vi "TfidfVectorizer.vi"(8 "error in":errorcluster caption="entrée d'erreur", 11 "TfidfVectorizer":T1={"encoding"="utf-8", "decode_error"="strict", "strip_accents"="None", "lowercase"=TRUE, "preprocessor"="None", "tokenizer"="None", "analyzer"="word", "stop_words"={"Type"="None", "list"=[]}, "token_pattern"="(?u)\\b\\w\\w+\\b", "ngram_range"={"min_n"=1, "max_n"=1}, "max_df"=1.0, "min_df"=1.0, "max_features"=-1, "vocabulary"={"Clé"=["None"], "Valeur"=[]}, "binary"=FALSE, "dtype"="float", "norm"="l2", "use_idf"=TRUE, "smooth_idf"=TRUE, "sublinear_tf"=FALSE} {"max_features" min=-1; "min_df" min=0.0 max=1.0; "max_df" min=0.0 max=1.0}) -> (0 "error out":errorcluster caption="sortie d'erreur", 3 "TfidfVectorizer.lvclass":refnum<class "TfidfVectorizer.lvclass">)   [LabVIEW 2020]
doc: "Convert a collection of raw documents to a matrix of TF-IDF features.\n\nEquivalent to CountVectorizer followed by TfidfTransformer.\n\nParameters :\n\n- encoding : str, default=’utf-8’\nIf bytes or files are given to analyze, this encoding is used to decode.\n\n- decode_error : {‘strict’, ‘ignore’, ‘replace’}, default=’strict’\nInstruction on what to do if a byte sequence is given to analyze that contains characters not of the given encoding. By default, it is ‘strict’, meaning that a UnicodeDecodeError will be raised. Other values are ‘ignore’ and ‘replace’.\n\n- strip_accents : {‘ascii’, ‘unicode’}, default=None\nRemove accents and perform other character normalization during the preprocessing step. ‘ascii’ is a fast method that only works on characters that have an direct ASCII mapping. ‘unicode’ is a slightly slower method that works on any characters. None (default) does nothing.\n\nBoth ‘ascii’ and ‘unicode’ use NFKD normalization from unicodedata.normalize.\n\n- lowercase : bool, default=True\nConvert all characters to lowercase before tokenizing.\n\n- preprocessor : callable, default=None\nOverride the preprocessing (string transformation) stage while preserving the tokenizing and n-grams generation steps. Only applies if analyzer is not callable.\n\n- tokenizer : callable, default=None\nOverride the string tokenization step while preserving the preprocessing and n-grams generation steps. Only applies if analyzer == 'word'.\n\n- analyzer : {‘word’, ‘char’, ‘char_wb’} or callable, default=’word’\nWhether the feature should be made of word or character n-grams. Option ‘char_wb’ creates character n-grams only from text inside word boundaries; n-grams at the edges of words are padded with space.\n\nIf a callable is passed it is used to extract the sequence of features out of the raw, unprocessed input.\n\n- stop_words : {‘english’}, list, default=None\nIf a string, it is passed to _check_stop_list and the appropriate stop list is returned. ‘english’ is currently the only supported string value. There are several known issues with ‘english’ and you should consider an alternative (see Using stop words).\n\nIf a list, that list is assumed to contain stop words, all of which will be removed from the resulting tokens. Only applies if analyzer == 'word'.\n\nIf None, no stop words will be used. max_df can be set to a value in the range [0.7, 1.0) to automatically detect and filter stop words based on intra corpus document frequency of terms.\n\n- token_pattern : str\nRegular expression denoting what constitutes a “token”, only used if analyzer == 'word'. The default regexp selects tokens of 2 or more alphanumeric characters (punctuation is completely ignored and always treated as a token separator).\n\n- ngram_range : tuple (min_n, max_n), default=(1, 1)\nThe lower and upper boundary of the range of n-values for different n-grams to be extracted. All values of n such that min_n <= n <= max_n will be used. For example an ngram_range of (1, 1) means only unigrams, (1, 2) means unigrams and bigrams, and (2, 2) means only bigrams. Only applies if analyzer is not callable.\n\n- max_df : float or int, default=1.0\nWhen building the vocabulary ignore terms that have a document frequency strictly higher than the given threshold (corpus-specific stop words). If float in range [0.0, 1.0], the parameter represents a proportion of documents, integer absolute counts. This parameter is ignored if vocabulary is not None.\n\n- min_df : float or int, default=1\nWhen building the vocabulary ignore terms that have a document frequency strictly lower than the given threshold. This value is also called cut-off in the literature. If float in range of [0.0, 1.0], the parameter represents a proportion of documents, integer absolute counts. This parameter is ignored if vocabulary is not None.\n\n- max_features : int, default=None\nIf not None, build a vocabulary that only consider the top max_features ordered by term frequency across the corpus.\n\nThis parameter is ignored if vocabulary is not None.\n\n- vocabulary : Mapping or iterable, default=None\nEither a Mapping (e.g., a dict) where keys are terms and values are indices in the feature matrix, or an iterable over terms. If not given, a vocabulary is determined from the input documents.\n\n- binary : bool, default=False\nIf True, all non-zero term counts are set to 1. This does not mean outputs will have only 0/1 values, only that the tf term in tf-idf is binary. (Set idf and normalization to False to get 0/1 outputs).\n\n- dtype : dtype, default=float64\nType of the matrix returned by fit_transform() or transform().\n\n- norm : {‘l1’, ‘l2’}, default=’l2’\nEach output row will have unit norm, either: * ‘l2’: Sum of squares of vector elements is 1. The cosine similarity between two vectors is their dot product when l2 norm has been applied. * ‘l1’: Sum of absolute values of vector elements is 1. See preprocessing.normalize.\n\n- use_idf : bool, default=True\nEnable inverse-document-frequency reweighting.\n\n- smooth_idf : bool, default=True\nSmooth idf weights by adding one to document frequencies, as if an extra document was seen containing every term in the collection exactly once. Prevents zero divisions.\n\n- sublinear_tf : bool, default=False\nApply sublinear tf scaling, i.e. replace tf with 1 + log(tf).\n\n\n\nMethods :"
uses:
  TfidfVectorizer.lvclass
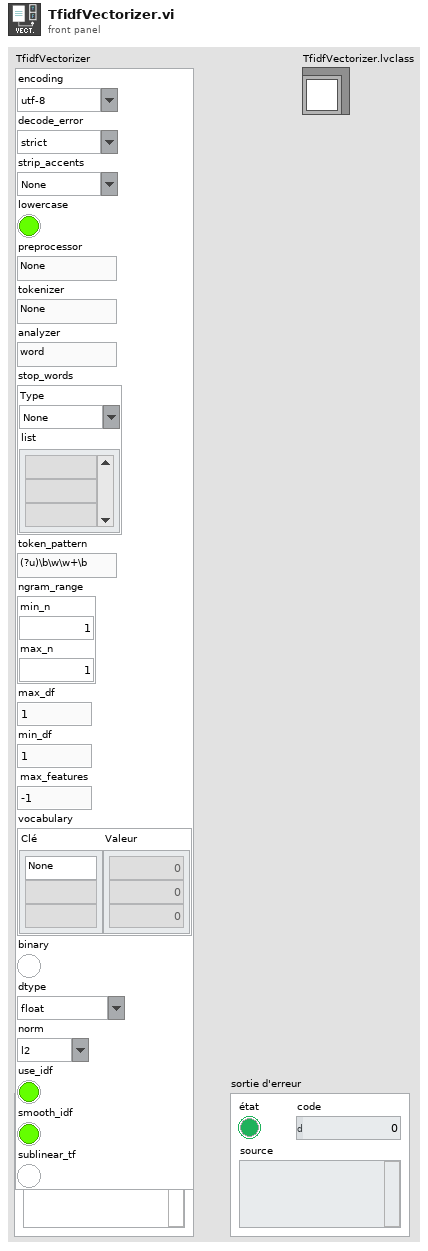
[diagram p1: front panel]
types:
  T1 = cluster{"encoding":string, "decode_error":string, "strip_accents":string, "lowercase":bool, "preprocessor":string, "tokenizer":string, "analyzer":string, "stop_words":cluster{"Type":string, "list":string[]}, "token_pattern":string, "ngram_range":cluster{"min_n":i32, "max_n":i32}, "max_df":dbl, "min_df":dbl, "max_features":i32, "vocabulary":cluster{"Clé":string[], "Valeur":i32[]}, "binary":bool, "dtype":string, "norm":string, "use_idf":bool, "smooth_idf":bool, "sublinear_tf":bool}
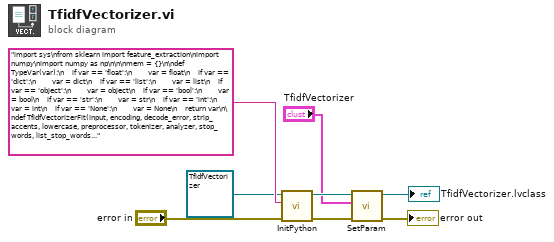
[diagram p0: block diagram]
diagram:
  n1 = call-dynamic "InitPython.vi"("error in (no error)"="error in", "Python Instruction"="import sys\nfrom sklearn import feature_extraction\nimport numpy\nimport numpy as np\n\n\nmem = {}\n\ndef TypeVar(var):\n    if var == 'float':\n        var = float\n    if var == 'dict':\n        var = dict\n    if var == 'list':\n        var = list\n    if var == 'object':\n        var = object\n    if var == 'bool':\n        var = bool\n    if var == 'str':\n        var = str\n    if var == 'int':\n        var = int\n    if var == 'None':\n        var = None\n    return var\n\ndef TfidfVectorizerFit(input, encoding, decode_error, strip_accents, lowercase, preprocessor, tokenizer, analyzer, stop_words, list_stop_words, token_pattern, min_n, max_n, max_df, min_df, max_features, vocabulary, binary, dtype, norm, use_idf, smooth_idf, sublinear_tf, X, doc):\n    X = eval(X)\n    dtype = TypeVar(dtype) \n    list_analyzer = ['word', 'char', 'char_wb']\n    if tokenizer == 'None' or tokenizer == '':\n        tokenizer = None\n    else:\n        tokenizer = eval(tokenizer)\n    if preprocessor == 'None' or preprocessor == '':\n        preprocessor = None\n    else:\n        preprocessor = eval(preprocessor)\n    if strip_accents == 'None':\n        strip_accents = None\n    if stop_words == 'None':\n        stop_words = None\n    elif stop_words == 'list':\n        stop_words = list_stop_words\n    else: \n        pass\n    if norm == 'None':\n        norm = None\n    if max_features == -1:\n        max_features = None\n    if vocabulary == 'None':\n        vocabulary = None\n    else:\n        vocabulary = eval(vocabulary)\n    if analyzer not in list_analyzer:\n        analyzer = eval(analyzer) \n    try:\n        TfidfVectorizer = feature_extraction.text.TfidfVectorizer(input, encoding, decode_error, strip_accents, lowercase, preprocessor, tokenizer, analyzer, stop_words, token_pattern, (min_n, max_n), max_df, min_df, max_features, vocabulary, binary, dtype, norm, use_idf, smooth_idf, sublinear_tf).fit(X)\n        mem['FitTfidfVectorizer'] = TfidfVectorizer\n        return str('OK')\n    except:\n        erreur = sys.exc_info()\n        typerr = u\"%s\" % (erreur[0])\n        typerr = typerr[typerr.find(\"'\")+1:typerr.rfind(\"'\")]\n        msgerr = u\"%s\" % (erreur[1])\n        message = str('/!\\\\ {0} : {1}'. format(typerr,msgerr))\n        return message \n\ndef TfidfVectorizerFitTransform(input, encoding, decode_error, strip_accents, lowercase, preprocessor, tokenizer, analyzer, stop_words, list_stop_words, token_pattern, min_n, max_n, max_df, min_df, max_features, vocabulary, binary, dtype, norm, use_idf, smooth_idf, sublinear_tf, X, doc):\n    X = eval(X)\n    dtype = TypeVar(dtype) \n    list_analyzer = ['word', 'char', 'char_wb']\n    if tokenizer == 'None' or tokenizer == '':\n        tokenizer = None\n    else:\n        tokenizer = eval(tokenizer)\n    if preprocessor == 'None' or preprocessor == '':\n        preprocessor = None\n    else:\n        preprocessor = eval(preprocessor)\n    if strip_accents == 'None':\n        strip_accents = None\n    if stop_words == 'None':\n        stop_words = None\n    elif stop_words == 'list':\n        stop_words = list_stop_words\n    else: \n        pass\n    if norm == 'None':\n        norm = None\n    if max_features == -1:\n        max_features = None\n    if vocabulary == 'None':\n        vocabulary = None\n    else:\n        vocabulary = eval(vocabulary)\n    if analyzer not in list_analyzer:\n        analyzer = eval(analyzer) \n    try:\n        TfidfVectorizer = feature_extraction.text.TfidfVectorizer(input, encoding, decode_error, strip_accents, lowercase, preprocessor, tokenizer, analyzer, stop_words, token_pattern, (min_n, max_n), max_df, min_df, max_features, vocabulary, binary, dtype, norm, use_idf, smooth_idf, sublinear_tf).fit_transform(X)\n        Mat = TfidfVectorizer.tocoo()\n        return str(list(zip(Mat.row, Mat.col, Mat.data)))\n    except:\n        erreur = sys.exc_info()\n        typerr = u\"%s\" % (erreur[0])\n        typerr = typerr[typerr.find(\"'\")+1:typerr.rfind(\"'\")]\n        msgerr = u\"%s\" % (erreur[1])\n        message = str('/!\\\\ {0} : {1}'. format(typerr,msgerr))\n        return message \n    \ndef TfidfVectorizerTransform(input, encoding, decode_error, strip_accents, lowercase, preprocessor, tokenizer, analyzer, stop_words, list_stop_words, token_pattern, min_n, max_n, max_df, min_df, max_features, vocabulary, binary, dtype, norm, use_idf, smooth_idf, sublinear_tf, X, doc):\n    X = eval(X)\n    dtype = TypeVar(dtype) \n    list_analyzer = ['word', 'char', 'char_wb']\n    if tokenizer == 'None' or tokenizer == '':\n        tokenizer = None\n    else:\n        tokenizer = eval(tokenizer)\n    if preprocessor == 'None' or preprocessor == '':\n        preprocessor = None\n    else:\n        preprocessor = eval(preprocessor)\n    if strip_accents == 'None':\n        strip_accents = None\n    if stop_words == 'None':\n        stop_words = None\n    elif stop_words == 'list':\n        stop_words = list_stop_words\n    else: \n        pass\n    if norm == 'None':\n        norm = None\n    if max_features == -1:\n        max_features = None\n    if vocabulary == 'None':\n        vocabulary = None\n    else:\n        vocabulary = eval(vocabulary)\n    if analyzer not in list_analyzer:\n        analyzer = eval(analyzer) \n    try:\n        TfidfVectorizer = mem['FitTfidfVectorizer'].transform(X)\n        Mat = TfidfVectorizer.tocoo()\n        return str(list(zip(Mat.row, Mat.col, Mat.data)))\n    except:\n        erreur = sys.exc_info()\n        typerr = u\"%s\" % (erreur[0])\n        typerr = typerr[typerr.find(\"'\")+1:typerr.rfind(\"'\")]\n        msgerr = u\"%s\" % (erreur[1])\n        message = str('/!\\\\ {0} : {1}'. format(typerr,msgerr))\n        return message\n    \ndef TfidfVectorizerDecode(input, encoding, decode_error, strip_accents, lowercase, preprocessor, tokenizer, analyzer, stop_words, list_stop_words, token_pattern, min_n, max_n, max_df, min_df, max_features, vocabulary, binary, dtype, norm, use_idf, smooth_idf, sublinear_tf, X, doc):\n    X = eval(X)\n    dtype = TypeVar(dtype) \n    list_analyzer = ['word', 'char', 'char_wb']\n    if tokenizer == 'None' or tokenizer == '':\n        tokenizer = None\n    else:\n        tokenizer = eval(tokenizer)\n    if preprocessor == 'None' or preprocessor == '':\n        preprocessor = None\n    else:\n        preprocessor = eval(preprocessor)\n    if strip_accents == 'None':\n        strip_accents = None\n    if stop_words == 'None':\n        stop_words = None\n    elif stop_words == 'list':\n        stop_words = list_stop_words\n    else: \n        pass\n    if norm == 'None':\n        norm = None\n    if max_features == -1:\n        max_features = None\n    if vocabulary == 'None':\n        vocabulary = None\n    else:\n        vocabulary = eval(vocabulary)\n    if analyzer not in list_analyzer:\n        analyzer = eval(analyzer) \n    try:\n        TfidfVectorizer = feature_extraction.text.TfidfVectorizer(input, encoding, decode_error, strip_accents, lowercase, preprocessor, tokenizer, analyzer, stop_words, token_pattern, (min_n, max_n), max_df, min_df, max_features, vocabulary, binary, dtype, norm, use_idf, smooth_idf, sublinear_tf).decode(doc)\n        return str(TfidfVectorizer)\n    except:\n        erreur = sys.exc_info()\n        typerr = u\"%s\" % (erreur[0])\n        typerr = typerr[typerr.find(\"'\")+1:typerr.rfind(\"'\")]\n        msgerr = u\"%s\" % (erreur[1])\n        message = str('/!\\\\ {0} : {1}'. format(typerr,msgerr))\n        return message\n    \ndef TfidfVectorizerFeatNames(input, encoding, decode_error, strip_accents, lowercase, preprocessor, tokenizer, analyzer, stop_words, list_stop_words, token_pattern, min_n, max_n, max_df, min_df, max_features, vocabulary, binary, dtype, norm, use_idf, smooth_idf, sublinear_tf, X, doc):\n    X = eval(X)\n    dtype = TypeVar(dtype) \n    list_analyzer = ['word', 'char', 'char_wb']\n    if tokenizer == 'None' or tokenizer == '':\n        tokenizer = None\n    else:\n        tokenizer = eval(tokenizer)\n    if preprocessor == 'None' or preprocessor == '':\n        preprocessor = None\n    else:\n        preprocessor = eval(preprocessor)\n    if strip_accents == 'None':\n        strip_accents = None\n    if stop_words == 'None':\n        stop_words = None\n    elif stop_words == 'list':\n        stop_words = list_stop_words\n    else: \n        pass\n    if norm == 'None':\n        norm = None\n    if max_features == -1:\n        max_features = None\n    if vocabulary == 'None':\n        vocabulary = None\n    else:\n        vocabulary = eval(vocabulary)\n    if analyzer not in list_analyzer:\n        analyzer = eval(analyzer) \n    try:\n        TfidfVectorizer = mem['FitTfidfVectorizer'].get_feature_names()\n        return str(TfidfVectorizer)\n    except:\n        erreur = sys.exc_info()\n        typerr = u\"%s\" % (erreur[0])\n        typerr = typerr[typerr.find(\"'\")+1:typerr.rfind(\"'\")]\n        msgerr = u\"%s\" % (erreur[1])\n        message = str('/!\\\\ {0} : {1}'. format(typerr,msgerr))\n        return message", "Scikit-learn en entrée"=refnum<class "TfidfVectorizer.lvclass"> refnum ("TfidfVectorizer.lvclass")) -> ("error out"=w4:errorcluster, "Scikit-learn en sortie"=w5:refnum<class "TfidfVectorizer.lvclass">)  [unwired: 7 in]
  n2 = call-dynamic "SetParam.vi"("error in (no error)"=w4, "TfidfVectorizer"="TfidfVectorizer", "TfidfVectorizer.lvclass"=w5) -> ("error out"=→"error out":errorcluster, "TfidfVectorizer.lvclass"=→"TfidfVectorizer.lvclass":refnum<class "TfidfVectorizer.lvclass">)  [unwired: 7 in]
